vi "Project1Labview.vi"() -> ()   [LabVIEW 2025]
panel:
  out "Numeric":dbl
  in  "Relative Humidity,%":dbl(slide) scale=0.0..10.0
  in  "Rsens,Kohm":dbl(slide) scale=0.0..10.0
  in  "V+,V":dbl(slide) scale=0.0..10.0
  in  "Vdiff,V":dbl(slide) scale=0.0..10.0
  in  "V_SCC,V":dbl(slide) scale=0.0..10.0
  out "Output (V)":dbl format="%04.3f"
  in  "stop":bool
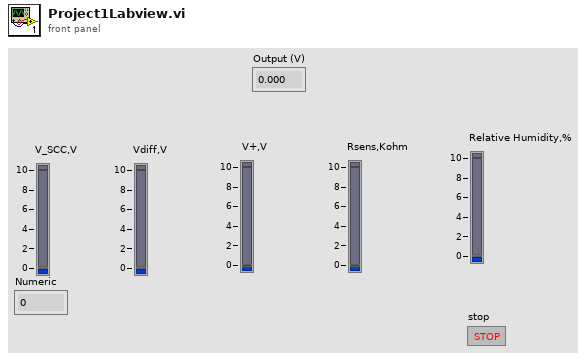
[diagram p1: front panel]
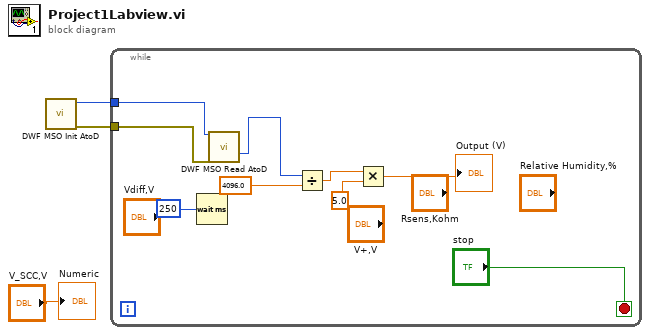
[diagram p0: block diagram]
diagram:
  n1 = call "DWF MSO Init AtoD.vi"() -> ("Error Out"=w2:errorcluster, "Instrument Handle Out"=w3:i32)  [unwired: 10 in]
  n2 = while {
    tunnel: w3 -> [w10]
    tunnel: w2 -> [w9]
    stop <- "stop" stop-if-true
    n3 = Wait (ms)(milliseconds to wait=u32 250 ("millisecond timer value")) -> ()  [unwired: 1 out]
    n4 = call "DWF MSO Read AtoD.vi"("Instrument Handle In AtoD"=w10, "Error In"=w9) -> ("AtoD"=w4:i16)  [unwired: 12 in, 1 out]
    n5 = Divide(x=w4, y=4096.0) -> (x/y=w6:dbl)
    n6 = Multiply(x=w6, y=5.0) -> (x*y=→"Output (V)":dbl)
  }
  "Numeric" <- "V_SCC,V"
